vi "tatambahan.vi"() -> ()   [LabVIEW 2015]
panel:
  in  "Numeric Control 2":u8
  out "Numeric Indicator":u8
  in  "Numeric Control":u8
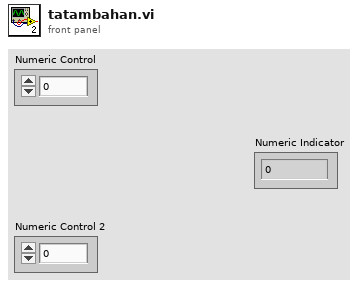
[diagram p1: front panel]
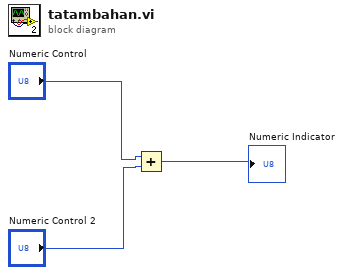
[diagram p0: block diagram]
diagram:
  n1 = Add(x="Numeric Control", y="Numeric Control 2") -> (x+y=→"Numeric Indicator":u8)
